vi "alignment_stand_alone.vi"() -> ()   [LabVIEW 2011]
uses:
  global_vars.vi
panel:
  in  "u16_choose_cam":u16(ring) items=[" HP Cam", "PixelLink Cam"]
  in  "dbl_shutter_value":dbl(slide)=0.036604516208171844 caption="Camera Shutter \n(PixelLink only)" min=0.001 max=1.0 scale=0.0..1.0
  out "Camera Stream":T1(plugin-control)
  in  "b_stream_window":bool caption="camera stream \nin extra window"
  in  "b_overlay_stream":bool caption="camera \noverlay"
  in  "i32_stream_OL_center_radius":dbl caption="center radius"
  in  "i32_stream_OL_#rings":i32=30 caption="#rings"
  in  "stream_OL_color":u32(colorbox)=16448250 caption="overlay color"
  in  "df_intial phase shift":dbl caption="intial phase shift"
  in  "i32_width":i32=500 caption="Width (Px)"
  in  "i32_height":i32=500 caption="Height (Px)"
  in  "df_#fringes":dbl=11.0 caption="#fringes"
  in  "save image of\ncamera stream":bool
  in  "File Path":path
  in  "b_flip_direction":bool
  in  "i32_fringe_OL_#rings":i32=20 caption="#rings"
  in  "i32_fringe_OL_center_radius":dbl caption="center radius"
  in  "overlay color":u32(colorbox)=16448250
  in  "b_align":bool caption="fringe \noverlay"
  in  "b_preview fringes":bool=TRUE caption="preview \nfringes"
  in  "b_fit_to_screen":bool
  in  "b_to_2nd_screen":bool
  in  "b_close":bool
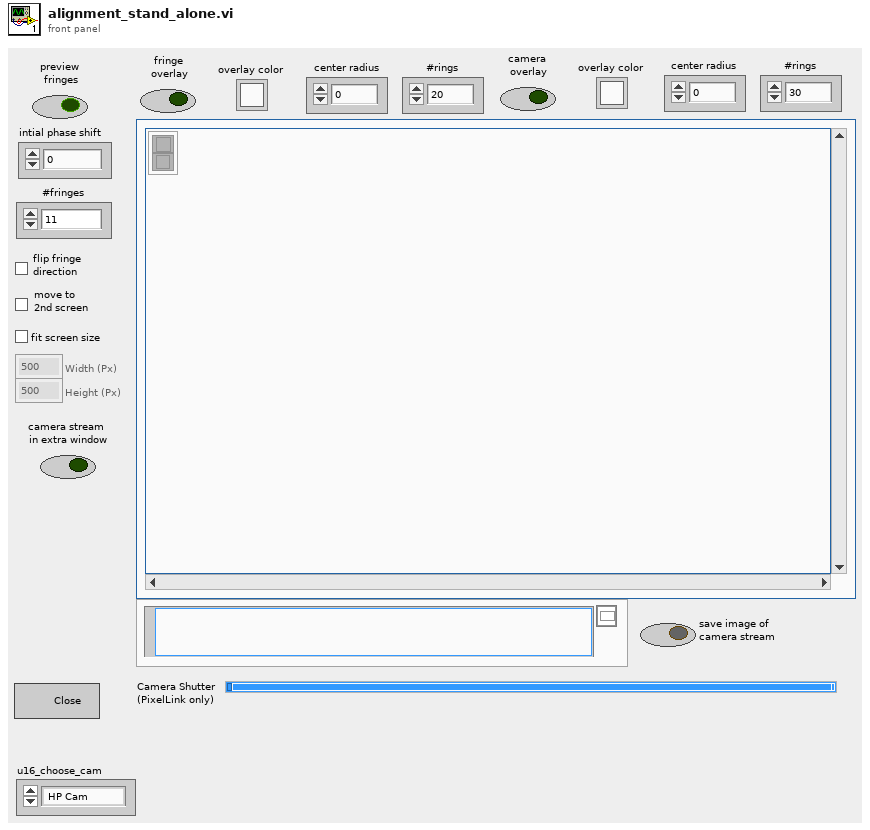
[diagram p1: front panel]
types:
  T1 = typedef "IMAQ Image.ctl" = refnum<image>
  T2 = enum8{"Enabled", "Disabled", "Disabled and Grayed Out"}
  T3 = cluster{"Numeric Control":i16, "Numeric Control":i16}
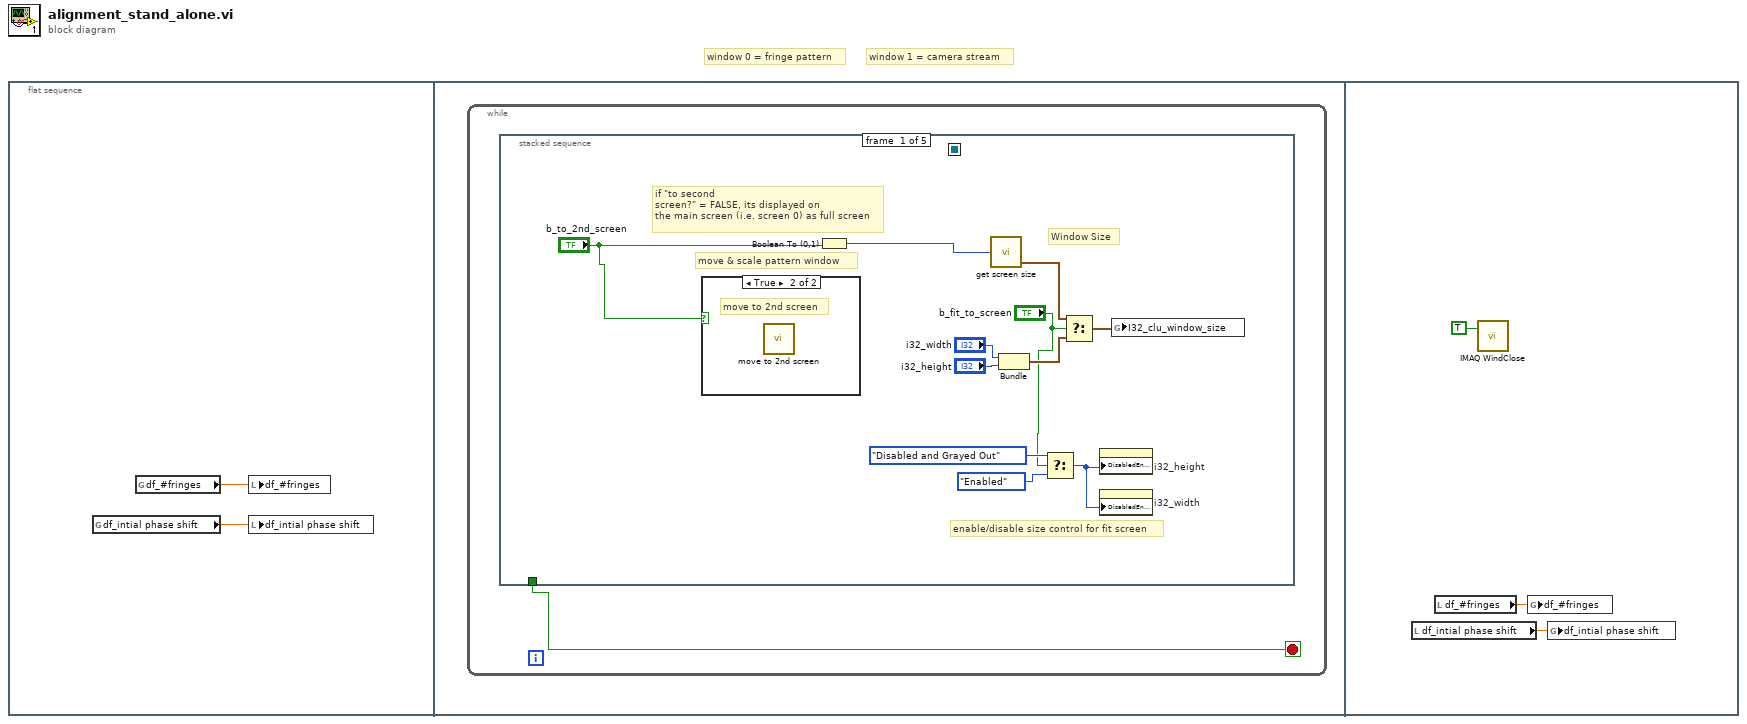
[diagram p0: block diagram]
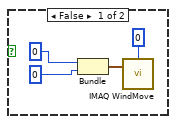
[diagram p2: hidden frame]
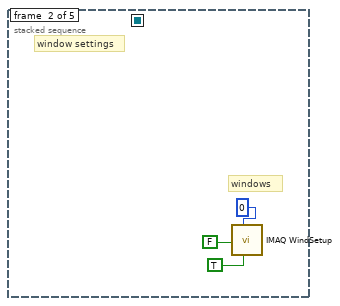
[diagram p3: hidden frame]
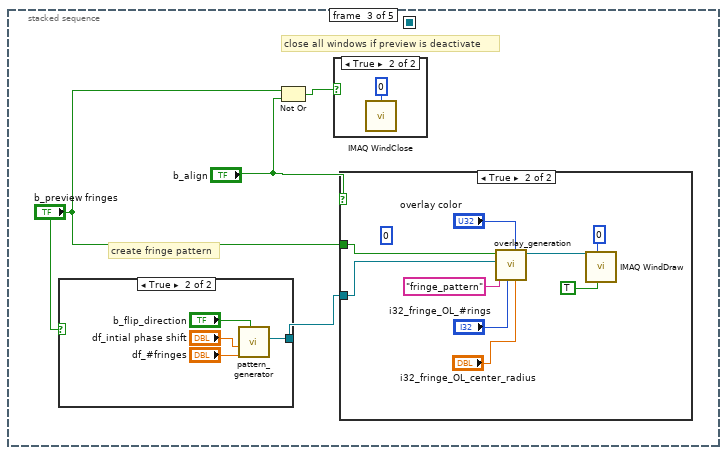
[diagram p4: hidden frame]
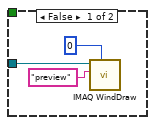
[diagram p6: hidden frame]
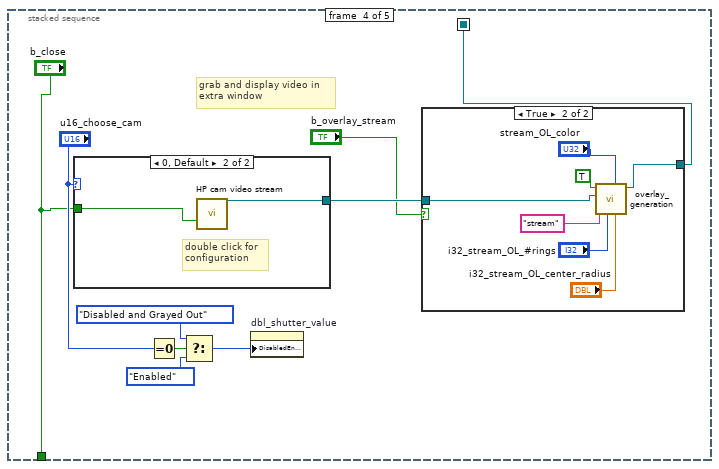
[diagram p8: hidden frame]
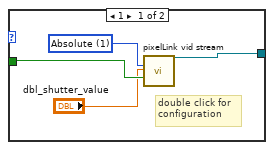
[diagram p9: hidden frame]
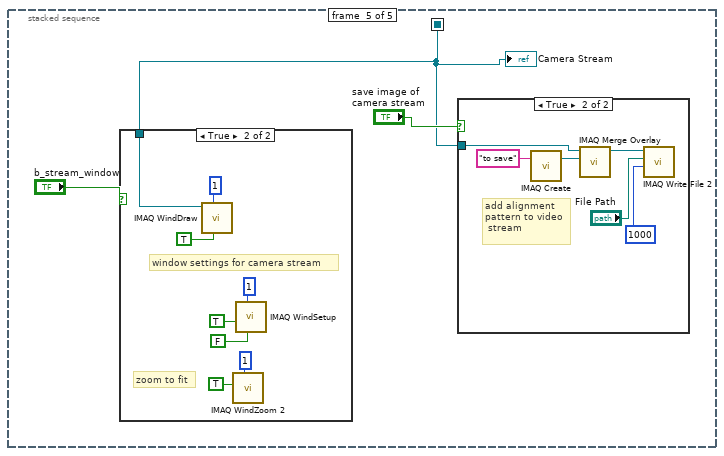
[diagram p11: hidden frame]
diagram:
  # "window 1 = camera stream"
  # "window 0 = fringe pattern"
  n1 = flat-sequence {
    frame #0 {
      n2 = global read "global_vars.vi" "df_intial phase shift"() -> (w1:dbl)
      n3 = global read "global_vars.vi" "df_#fringes"() -> (w2:dbl)
      n4 = local write "df_#fringes"(w2) -> ()
      n5 = local write "df_intial phase shift"(w1) -> ()
    }
    frame #1 {
      n6 = while {
        stop <- w3 stop-if-true
        n7 = stacked-sequence {
          seq-local: [_ _ _ w51 _] -> [_ _ _ _ w66]
          tunnel: [_ _ _ "b_close" _] -> w3
          frame #0 {
            # "enable/disable size control for fit screen"
            # "if \"to second \nscreen?\" = FALSE, its displayed on \nthe main screen (i.e. screen 0) as full screen"
            # "Window Size"
            # "move & scale pattern window"
            n8 = case shown="True" "b_to_2nd_screen" {
              frame False {
                n9 = Bundle(0, 0) -> (w18:cluster{i32, i32})  [unwired: 1 in]
                n10 = call "IMAQ WindMove"("Window Number (0...15)"=0, "Coordinates (screen)"=w18) -> ()  [unwired: 3 in, 2 out]
              }
              frame True {
                # "move to 2nd screen"
                n11 = call "move to 2nd screen.vi"() -> ()  [unwired: 12 in]
              }
            }
            n12 = Boolean To (0,1)(Boolean="b_to_2nd_screen") -> (0, 1=w14:i16)
            n13 = call "get screen size.vi"("screen"=w14) -> ("wind size (width/height)"=w13:T3)  [unwired: 2 in, 2 out]
            n14 = Bundle("i32_width"="i32_width", "i32_height"="i32_height") -> (w11:cluster{"i32_width":i32, "i32_height":i32})  [unwired: 1 in]
            n15 = Select(t=T2."Disabled and Grayed Out" ("Disabled"), s="b_fit_to_screen", f=T2."Enabled" ("Disabled")) -> (s? t:f=w4:T2)
            n16 = Select(t=w13, s="b_fit_to_screen", f=w11) -> (s? t:f=w12:cluster{"i32_width":i32, "i32_height":i32})
            n17 = property on="i32_height" class="DigNum (strict)"("DisabledEnum"=w4) -> ()  [unwired: 2 in, 2 out]
            n18 = property on="i32_width" class="DigNum (strict)"("DisabledEnum"=w4) -> ()  [unwired: 2 in, 2 out]
            n19 = global write "global_vars.vi" "I32_clu_window_size"(w12) -> ()
          }
          frame #1 {
            # "window settings"
            # "windows"
            n20 = call "IMAQ WindSetup"("Window is floating? (No)"=TRUE, "Window Number (0...15)"=0, "Window has title bar? (Yes)"=FALSE) -> ()  [unwired: 8 in, 1 out]
          }
          frame #2 {
            # "close all windows if preview is deactivate"
            # "create fringe pattern"
            n21 = case shown="True" "b_preview fringes" {
              tunnel: [_ w42] -> w22
              frame False {
              }
              frame True {
                n22 = call "pattern_generator.vi"("flip direction"="b_flip_direction", "fringe number"="df_#fringes", "phase"="df_intial phase shift") -> ("fringe pattern"=w42:T1)  [unwired: 7 in, 1 out]
              }
            }
            n23 = Not Or(1:"b_align", 2:"b_preview fringes") -> (0:w23:bool)
            n24 = case shown="True" w23 {
              frame False {
              }
              frame True {
                n25 = call "IMAQ WindClose"("Window Number (0...15)"=0) -> ()  [unwired: 5 in, 1 out]
              }
            }
            n26 = case shown="True" "b_align" {
              tunnel: w22 -> [w28 w38]
              tunnel: "b_preview fringes" -> [_ w37]
              frame False {
                n27 = call "IMAQ WindDraw"("Window Number (0...15)"=0, "Title"="preview", "Image"=w28) -> ()  [unwired: 7 in, 2 out]
              }
              frame True {
                (unwired) 0 ("Window Number (0...15)")
                n28 = call "overlay_generation.vi"("center radius"="i32_fringe_OL_center_radius", "Color"="overlay color", "number of rings"="i32_fringe_OL_#rings", "Title"="fringe_pattern", "Image Src"=w38, "fringe preview on"=w37) -> ("stream_overlay_out"=w30:T1)  [unwired: 5 in]
                n29 = call "IMAQ WindDraw"("Resize to Image Size? (Y)"=TRUE, "Window Number (0...15)"=0, "Image"=w30) -> ()  [unwired: 7 in, 2 out]
              }
            }
          }
          frame #3 {
            # "grab and display video in \nextra window"
            n30 = case shown="0, Default" "u16_choose_cam" {
              tunnel: [w55 w57] -> w50
              tunnel: "b_close" -> [w54 w56]
              frame 1 {
                w53 = u32 1 items=["Absolute"=1, "Auto"=3, "Relative"=0, "One Push"=4, "Ignored"=5] ("Shutter::Mode")
                # "double click for\nconfiguration"
                n31 = call "pixelLink vid stream"("Shutter::Mode"=w53, "Shutter::Value"="dbl_shutter_value", "Stop (F)"=w54) -> ("Image Out"=w55:T1)  [unwired: 20 in, 4 out]
              }
              frame 0, Default {
                # "double click for\nconfiguration"
                n32 = call "HP cam video stream"("Stop (F)"=w56) -> ("Image Out"=w57:T1)  [unwired: 22 in, 4 out]
              }
            }
            n33 = Equal To 0?(x="u16_choose_cam") -> (x = 0?=w44:bool)
            n34 = Select(t=T2."Disabled and Grayed Out" ("Disabled"), s=w44, f=T2."Enabled" ("Disabled")) -> (s? t:f=w47:T2)
            n35 = property on="dbl_shutter_value" class="Slide (strict)"("DisabledEnum"=w47) -> ()  [unwired: 2 in, 2 out]
            n36 = case shown="True" "b_overlay_stream" {
              tunnel: w50 -> [w58 w60]
              tunnel: [w58 w59] -> w51
              frame False {
              }
              frame True {
                n37 = call "overlay_generation.vi"("center radius"="i32_stream_OL_center_radius", "Color"="stream_OL_color", "number of rings"="i32_stream_OL_#rings", "Title"="stream", "Image Src"=w60, "fringe preview on"=TRUE) -> ("stream_overlay_out"=w59:T1)  [unwired: 5 in]
              }
            }
          }
          frame #4 {
            n38 = case shown="True" "b_stream_window" {
              tunnel: w66 -> [_ w74]
              frame False {
              }
              frame True {
                # "zoom to fit"
                # "window settings for camera stream"
                n39 = call "IMAQ WindDraw"("Resize to Image Size? (Y)"=TRUE, "Window Number (0...15)"=1, "Image"=w74) -> ()  [unwired: 7 in, 2 out]
                n40 = call "IMAQ WindZoom 2"("Window Number (0...15)"=1, "Zoom to Fit? (False)"=TRUE) -> ()  [unwired: 6 in, 4 out]
                n41 = call "IMAQ WindSetup"("Window is floating? (No)"=FALSE ("b_floating"), "Window Number (0...15)"=1, "Window has title bar? (Yes)"=TRUE ("b_title_bar")) -> ()  [unwired: 8 in, 1 out]
              }
            }
            n42 = case shown="True" "save image of\ncamera stream" {
              tunnel: w66 -> [_ w78]
              frame False {
              }
              frame True {
                # "add alignment\npattern to video\n stream"
                n43 = call "IMAQ Create"("Image Name"="to save") -> ("New Image"=w80:T1)  [unwired: 3 in, 2 out]
                n44 = call "IMAQ Merge Overlay"("Image Dst"=w80, "Image Src"=w78) -> ("Image Dst Out"=w77:T1)  [unwired: 8 in, 1 out]
                n45 = call-poly "IMAQ Write File 2"("Image Quality"=u32 1000, "File Path"="File Path", "Image"=w77) -> ()  [unwired: 7 in, 2 out]
              }
            }
            "Camera Stream" <- w66
          }
        }
      }
    }
    frame #2 {
      n46 = local read "df_intial phase shift"() -> (w85:dbl)
      n47 = local read "df_#fringes"() -> (w84:dbl)
      n48 = call "IMAQ WindClose"("Close All Windows (False)"=TRUE) -> ()  [unwired: 5 in, 1 out]
      n49 = global write "global_vars.vi" "df_#fringes"(w84) -> ()
      n50 = global write "global_vars.vi" "df_intial phase shift"(w85) -> ()
    }
  }
